vi "TA_Plot_Kinetics.vi"(10 "DeltaA (mOD)":dbl[][](array[numeric])=array214x154[32956 elements], 11 "Time (ps)":dbl[](array[numeric])=[-8.0, -7.0, -6.0, -5.0, -4.0, -3.0, -2.0, -1.0, -0.0, -0.0, -0.0, -0.0, -0.0, -0.0, -0.0, -0.0, -0.0, -0.0, -0.0, -0.0, -0.0, -0.0, -0.0, -0.0, 0.0, 0.0, 0.0, 0.0, 0.0, 0.0, 0.0, 0.0, 0.0, 0.0, 0.0, 0.0, 0.0, 0.0, 0.0, 0.0, 0.0, 0.0, 0.0, 0.0, 1.0, 1.0, 1.0, 1.0, 1.0, 1.0, 1.0, 1.0, 1.0, 1.0, 1.0, 1.0, 2.0, 2.0, 2.0, 2.0, 2.0, 2.0, 3.0, 3.0, 3.0, 3.0, 3.0, 4.0, 4.0, 4.0, 4.0, 4.0, 5.0, 5.0, 5.0, 6.0, 6.0, 7.0, 7.0, 8.0, 8.0, 9.0, 9.0, 10.0, 11.0, 12.0, 13.0, 14.0, 15.0, 16.0, 17.0, 18.0, 19.0, 20.0, 22.0, 24.0, 26.0, 28.0, 30.0, 32.0, 34.0, 36.0, 38.0, 40.0, 42.0, 44.0, 46.0, 48.0, 50.0, 55.0, 60.0, 65.0, 70.0, 75.0, 80.0, 85.0, 90.0, 95.0, 100.0, 110.0, 120.0, 130.0, 140.0, 150.0, 160.0, 170.0, 180.0, 190.0, 200.0, 220.0, 240.0, 260.0, 280.0, 300.0, 320.0, 340.0, 360.0, 380.0, 400.0, 420.0, 440.0, 460.0, 480.0, 500.0, 550.0, 600.0, 650.0, 700.0, 750.0, 800.0, 850.0, 900.0, 950.0, 1000.0]) -> (3 "TA Kinetics":cluster{"Array":dbl[], "Array 2":dbl[]}[](graph))   [LabVIEW 2025]
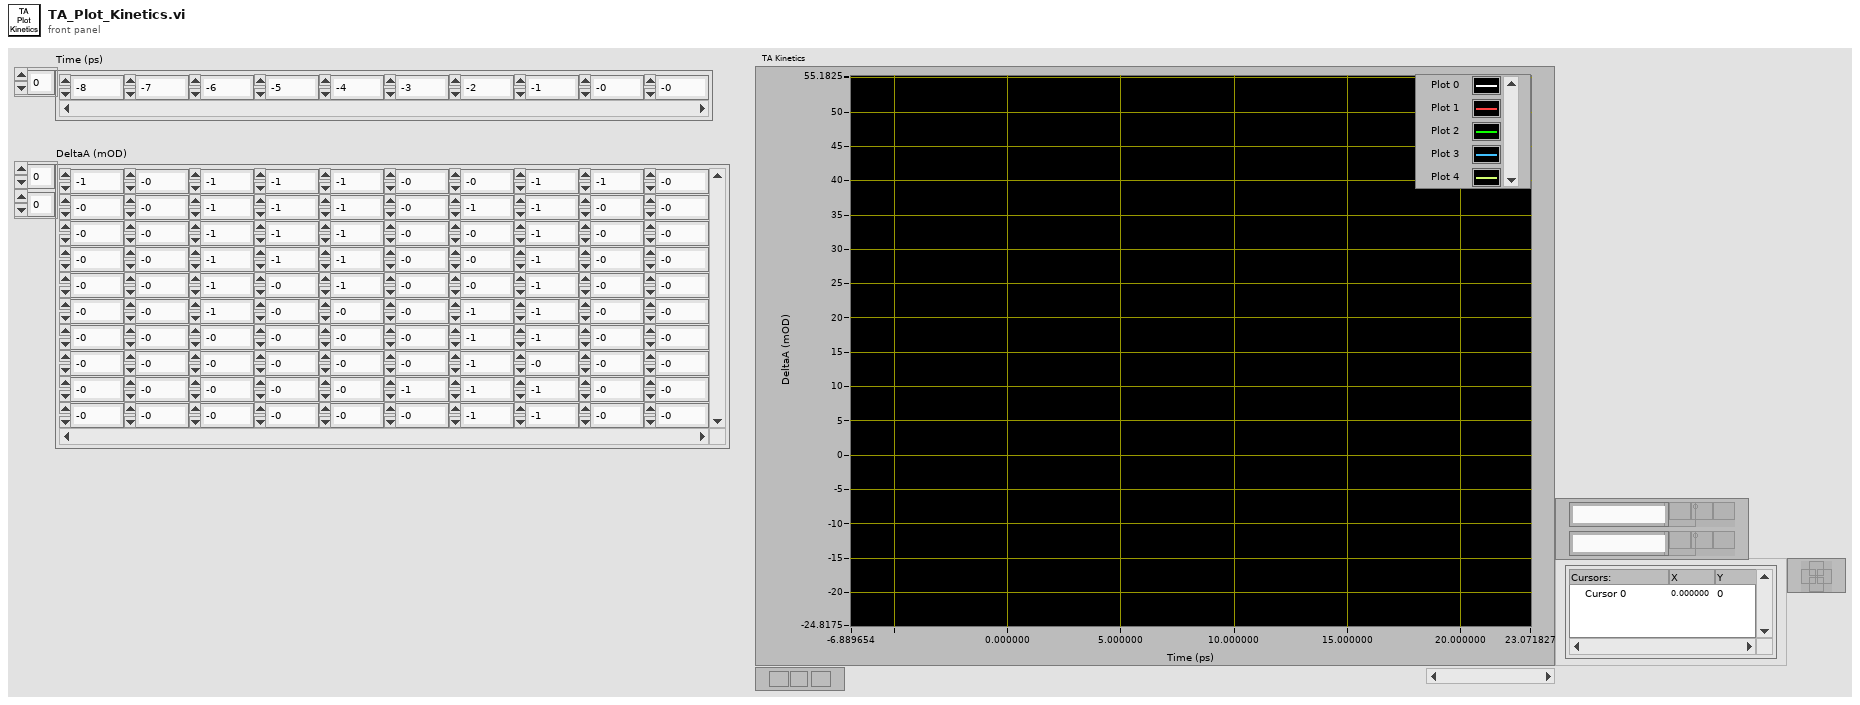
[diagram p1: front panel]
types:
  T1 = cluster{"Time (ps)":dbl[], "DeltaA (mOD)":dbl[]}[]
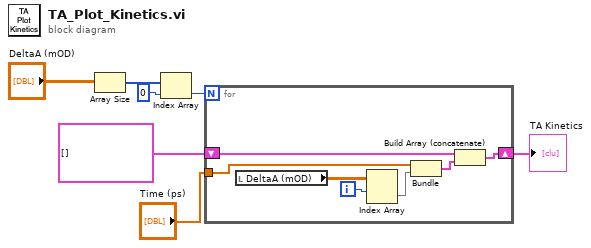
[diagram p0: block diagram]
diagram:
  n1 = Array Size(array="DeltaA (mOD)") -> (size(s)=w4:i32[])
  n2 = Index Array(array=w4, index=0) -> (element=w5:i32)
  n3 = for {
    N: w5 -> [_]
    tunnel: "Time (ps)" -> [w14]
    shift-right: [w9] -> w1
    shift-left: cluster{"Array":dbl[], "Array 2":dbl[]}[] [] ("Array") -> [w8]
    i -> [w13]
    n4 = local read "DeltaA (mOD)"() -> (w11:dbl[][])
    n5 = Index Array(array=w11, index (row)=w13) -> (element=w12:dbl[])  [unwired: 1 in]
    n6 = Bundle("Time (ps)"=w14, "DeltaA (mOD)"=w12) -> (w10:cluster{"Time (ps)":dbl[], "DeltaA (mOD)":dbl[]})  [unwired: 1 in]
    n7 = Build Array (concatenate)(w8, w10) -> (w9:T1)
  }
  "TA Kinetics" <- w1
